vi "Main.vi"() -> ()   [LabVIEW 2011]
panel:
  out "number (0 to 1)":dbl
  in  "stop":bool
  in  "OK Button":bool
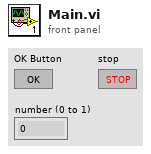
[diagram p1: front panel]
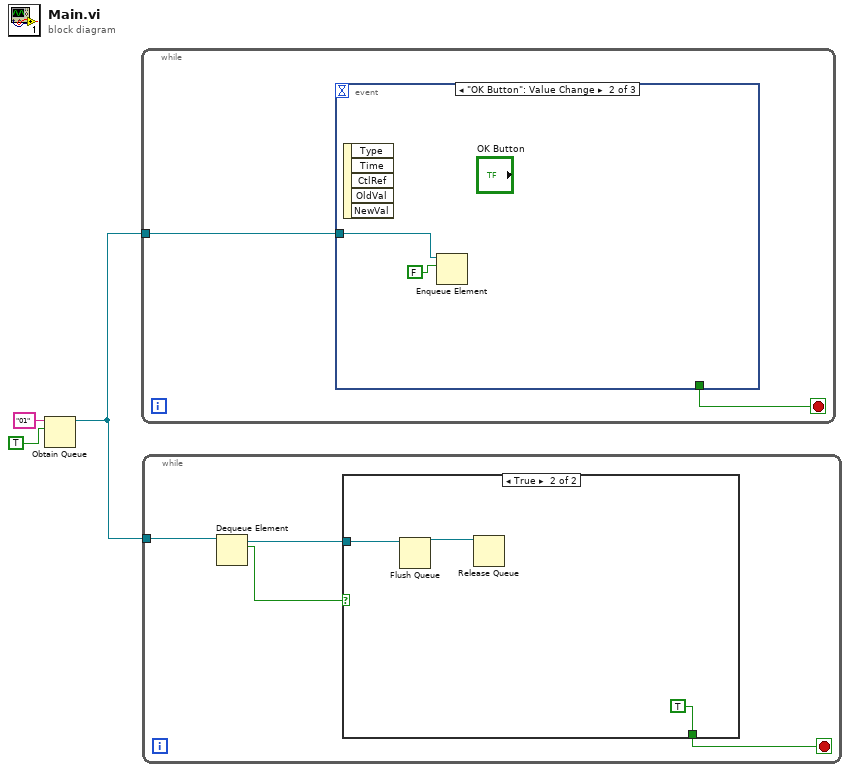
[diagram p0: block diagram]
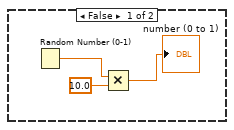
[diagram p2: hidden frame]
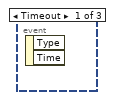
[diagram p3: hidden frame]
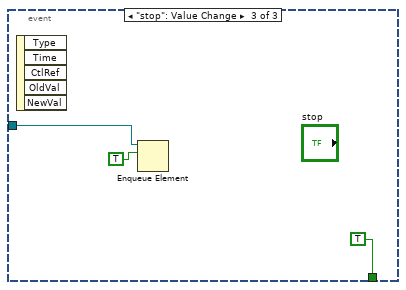
[diagram p4: hidden frame]
diagram:
  n1 = Obtain Queue(name (unnamed)="01", element data type=TRUE) -> (queue out=w1:refnum<queue>)  [unwired: 3 in, 2 out]
  n2 = while {
    tunnel: w1 -> [w5]
    stop <- w4 stop-if-true
    n3 = event shown="[1] \"OK Button\": Value Change" {
      selector: _ -> [_ _ _]
      dyn-events: _ -> [_ _ _]
      timeout: _ -> [_ _ _]
      tunnel: w5 -> [_ w6 w10]
      tunnel: [_ _ TRUE] -> w4
      event Timeout {
        n4 = event-data() -> ()  [unwired: 1 in, 2 out]
      }
      event "OK Button": Value Change {
        n5 = event-data() -> ()  [unwired: 1 in, 5 out]
        n6 = Enqueue Element(queue=w6, element=FALSE) -> ()  [unwired: 2 in, 3 out]
      }
      event "stop": Value Change {
        n7 = event-data() -> ()  [unwired: 1 in, 5 out]
        n8 = Enqueue Element(queue=w10, element=TRUE) -> ()  [unwired: 2 in, 3 out]
      }
    }
  }
  n9 = while {
    tunnel: w1 -> [w14]
    stop <- w12 stop-if-true
    n10 = Dequeue Element(queue=w14) -> (queue out=w11:refnum<queue>, element=w13:bool)  [unwired: 2 in, 2 out]
    n11 = case shown="True" w13 {
      tunnel: [_ TRUE] -> w12
      tunnel: w11 -> [_ w19]
      frame False {
        n12 = Random Number (0-1)() -> (number: 0 to 1=w17:dbl)
        n13 = Multiply(x=w17, y=10.0) -> (x*y=→"number (0 to 1)":dbl)
      }
      frame True {
        n14 = Flush Queue(queue=w19) -> (queue out=w18:refnum<queue>)  [unwired: 1 in, 2 out]
        n15 = Release Queue(queue=w18) -> ()  [unwired: 2 in, 3 out]
      }
    }
  }
